vi "Boiler System Open.vi"(8 "error in (no error)":errorcluster) -> (0 "error out":errorcluster, 2 "Notifiers":T2, 3 "Message Queues out":T1, 5 "User Event - Stop":refnum<user-event>, 7 "Stop Event Registration Refnum":refnum<event-registration>)   [LabVIEW 2015]
uses:
  Notifires.ctl
  Notifiers.ctl
  Message Queue/All Message Queues.ctl
  Message Queue/Message Cluster.ctl
  User Event - Stop/User Event - Stop.lvlib
  Message Queue/Message Queue.lvlib
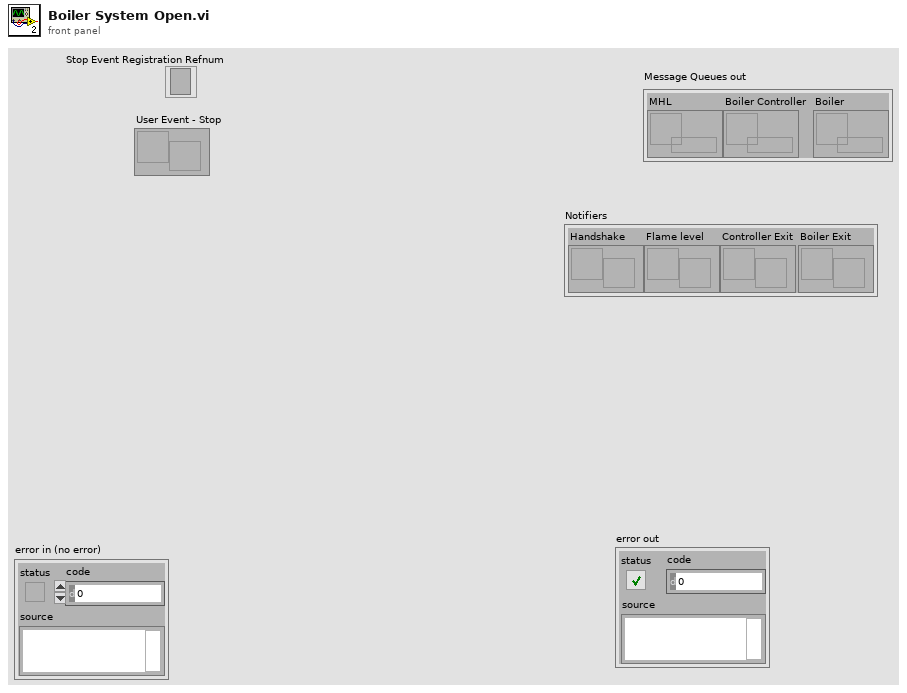
[diagram p1: front panel]
types:
  T1 = typedef "Message Queue.lvlib/All Message Queues.ctl" = cluster{"MHL":refnum<queue>, "Boiler Controller":refnum<queue>, "Boiler":refnum<queue>}
  T2 = typedef "Notifires.ctl" = cluster{"Handshake":refnum<notifier>, "Flame level":T3, "Controller Exit":refnum<notifier>, "Boiler Exit":refnum<notifier>}
  T3 = typedef "Notifiers.ctl" = refnum<notifier>
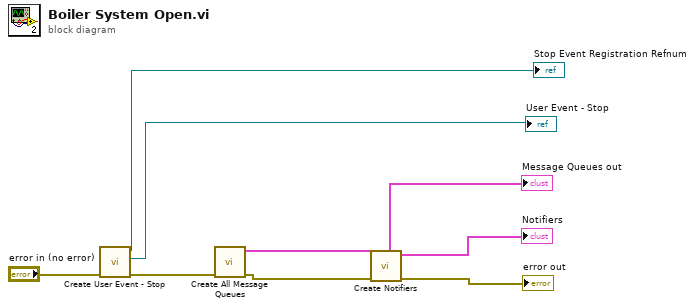
[diagram p0: block diagram]
diagram:
  n1 = call "Create User Event - Stop.vi"("error in (no error)"="error in (no error)") -> ("error out"=w7:errorcluster, "User Event - Stop"=→"User Event - Stop":refnum<user-event>, "Stop Event Registration Refnum"=→"Stop Event Registration Refnum":refnum<event-registration>)  [unwired: 8 in]
  n2 = call "Create All Message Queues.vi"("error in"=w7) -> ("error out"=w6:errorcluster, "Message Queues out"=→"Message Queues out":T1)  [unwired: 9 in]
  n3 = call "Create Notifiers.vi"("error in (no error)"=w6) -> ("error out"=→"error out":errorcluster, "Notifiers"=→"Notifiers":T2)  [unwired: 9 in]
